vi "AlignMini.vi"() -> ()   [LabVIEW 2019]
uses:
  <vilib>/userDefined/High Color/IMAQdx.ctl
  <vilib>/vision/driver/NI_Vision_Acquisition_Software.lvlib
  <vilib>/vision/NI_Vision_Development_Module.lvlib
panel:
  in  "Second Fiducial in View?":bool
  out "Image Out":T1(plugin-control)
  in  "Fiducial 1":bool
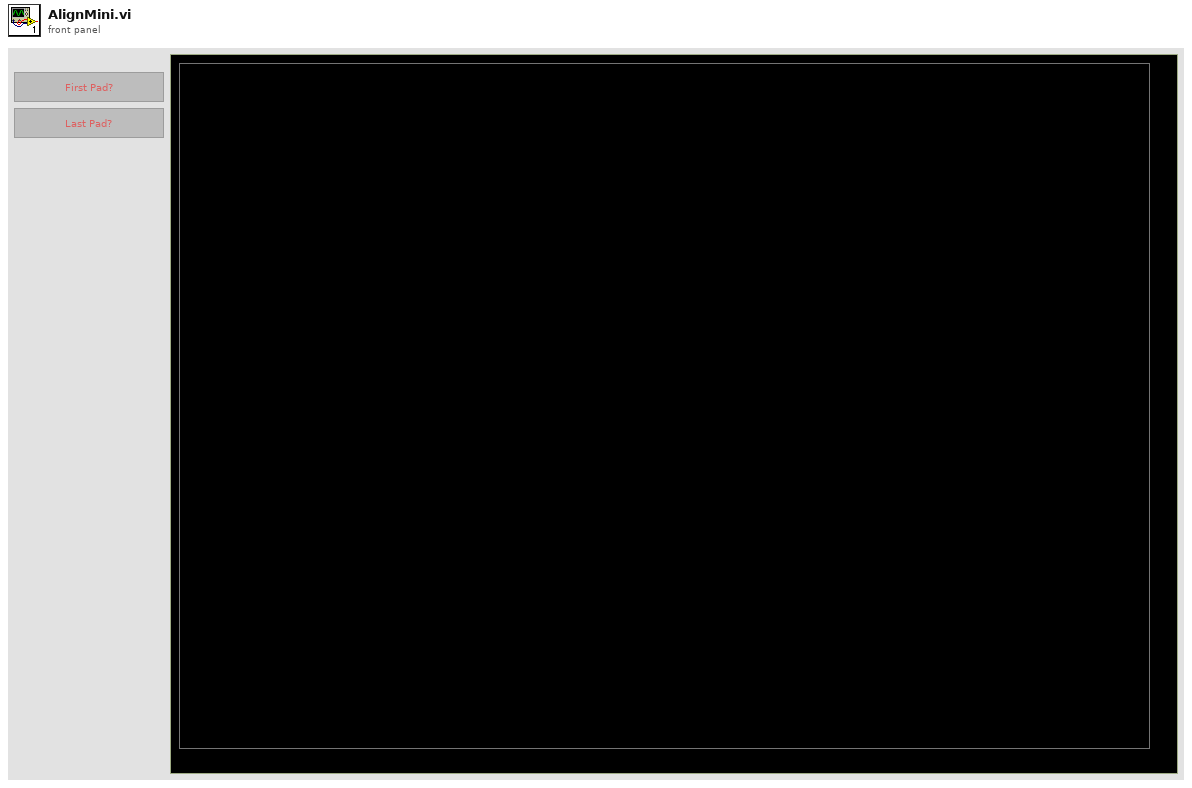
[diagram p1: front panel]
types:
  T1 = typedef "IMAQ Image.ctl" = refnum<image>
  T2 = enum8{"Enabled", "Disabled", "Disabled and Grayed Out"}
  T3 = typedef "Image Type" = u32
  T4 = typedef "IMAQdx.ctl" = refnum<k21>
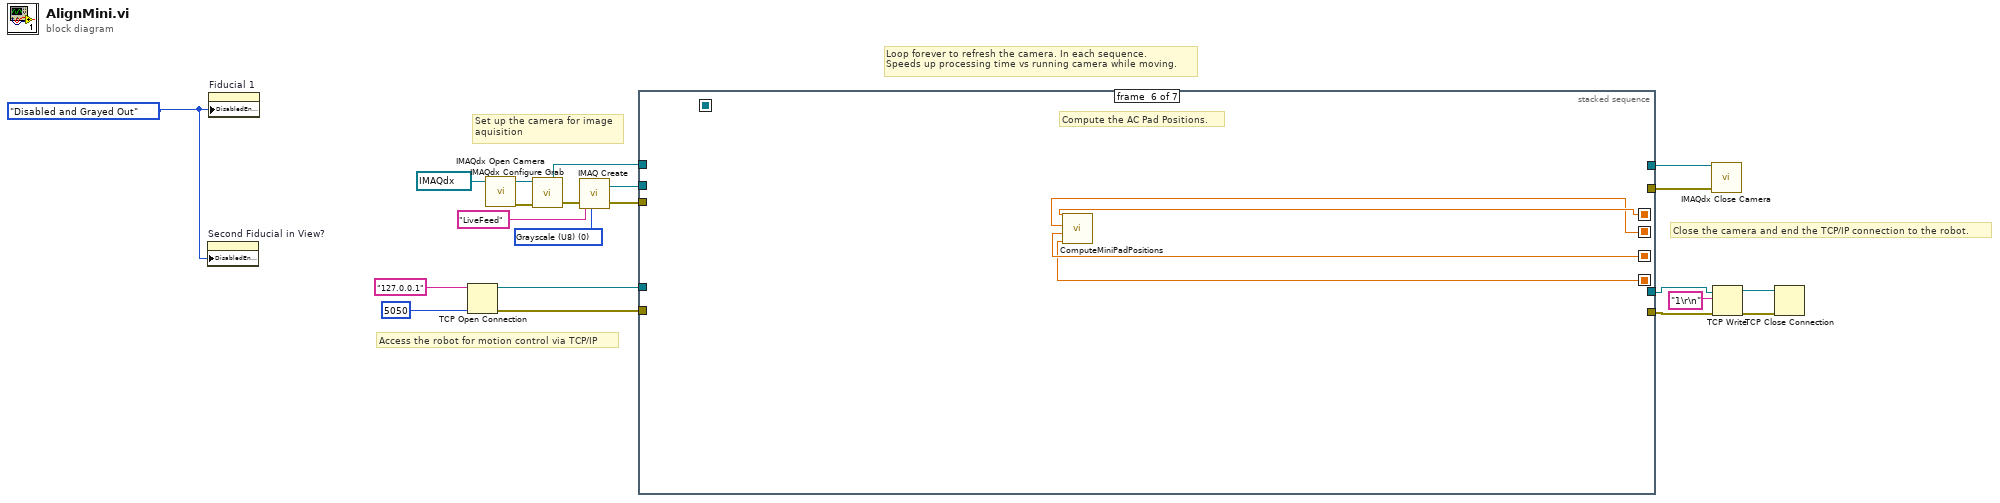
[diagram p0: block diagram]
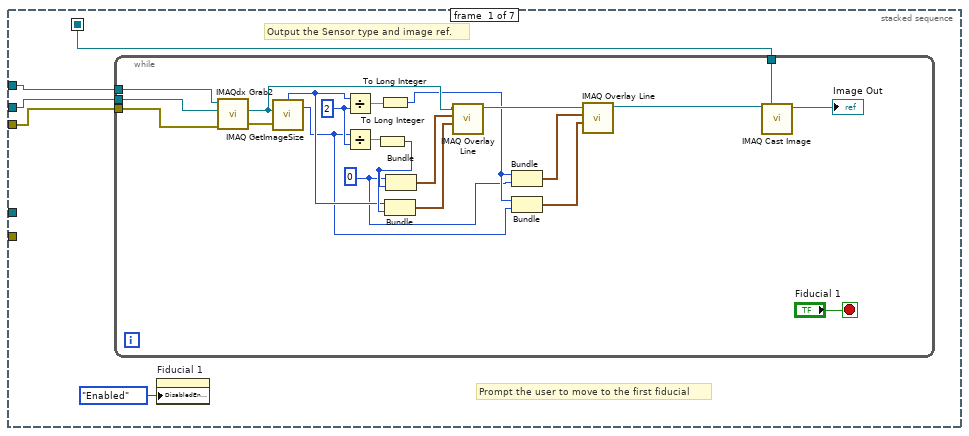
[diagram p2: hidden frame]
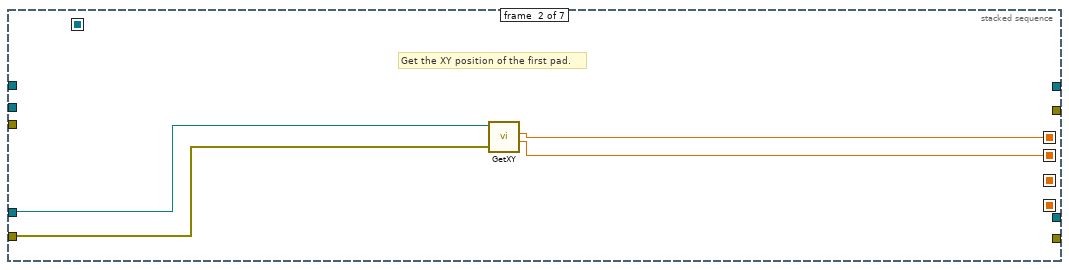
[diagram p3: hidden frame]
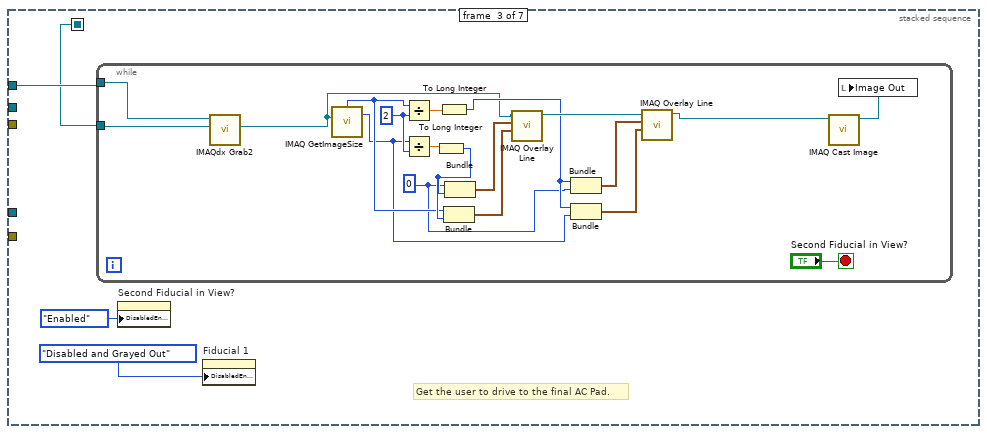
[diagram p4: hidden frame]
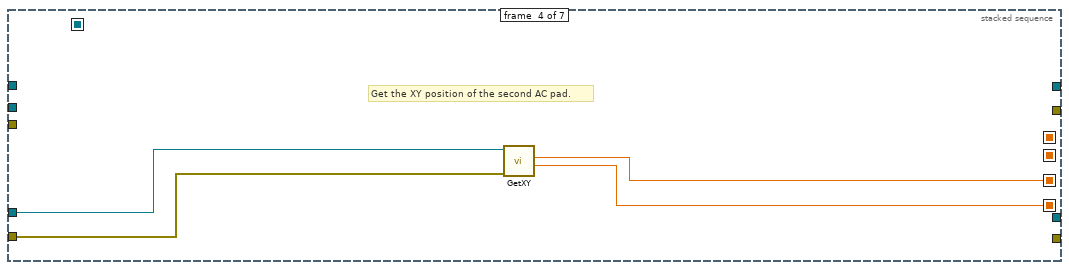
[diagram p5: hidden frame]
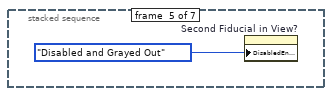
[diagram p6: hidden frame]
diagram:
  w1 = T2."Disabled and Grayed Out" ("Disabled")
  w11 = T3 0 items=["Grayscale (U8)", "Grayscale (I16)", "Grayscale (SGL)", "Complex (CSG)", "RGB (U32)", "HSL (U32)", "RGB (U64)", "Grayscale (U16)"] ("Image Type")
  # "Close the camera and end the TCP/IP connection to the robot."
  # "Access the robot for motion control via TCP/IP"
  # "Loop forever to refresh the camera. In each sequence. \nSpeeds up processing time vs running camera while moving."
  # "Set up the camera for image \naquisition"
  n1 = property on="Second Fiducial in View?" class="Bool"("DisabledEnum"=w1) -> ()  [unwired: 2 in, 2 out]
  n2 = property on="Fiducial 1" class="Bool"("DisabledEnum"=w1) -> ()  [unwired: 2 in, 2 out]
  n3 = TCP Open Connection(address="127.0.0.1", remote port or service name=u16 5050) -> (connection ID=w8:refnum<k5>, error out=w7:errorcluster)  [unwired: 3 in]
  n4 = call <vilib>:"IMAQdx Open Camera.vi"("Session In"=T4 "cam0") -> ("error out"=w19:errorcluster, "Session Out"=w20:T4)  [unwired: 9 in]
  n5 = call <vilib>:"IMAQdx Configure Grab.vi"("error in"=w19, "Session In"=w20) -> ("error out"=w17:errorcluster, "Session Out"=w16:T4)  [unwired: 8 in]
  n6 = call "IMAQ Create"("Image Name"="LiveFeed", "Image Type"=w11, "error in (no error)"=w17) -> ("New Image"=w15:T1, "error out"=w14:errorcluster)  [unwired: 2 in]
  n7 = stacked-sequence {
    seq-local: [w23 _ _ _ _ _ _] -> [_ _ w54 _ _ _ _]
    seq-local: [_ _ _ w76 _ _ _] -> [_ _ _ _ _ w81 _]
    seq-local: [_ _ _ w75 _ _ _] -> [_ _ _ _ _ w80 _]
    seq-local: [_ w49 _ _ _ _ _] -> [_ _ _ _ _ w83 _]
    seq-local: [_ w48 _ _ _ _ _] -> [_ _ _ _ _ w82 _]
    tunnel: w16 -> [w26 _ w55 _ _ _ w86]
    tunnel: w15 -> [w25 _ _ _ _ _ _]
    tunnel: w14 -> [w24 _ _ _ _ _ w87]
    tunnel: [_ _ _ _ _ _ w87] -> w13
    tunnel: [_ _ _ _ _ _ w86] -> w12
    tunnel: w8 -> [_ w51 _ w78 _ _ w85]
    tunnel: [_ _ _ _ _ _ w85] -> w5
    tunnel: [_ _ _ _ _ _ w84] -> w6
    tunnel: w7 -> [_ w50 _ w77 _ _ w84]
    frame #0 {
      # "Output the Sensor type and image ref."
      # "Prompt the user to move to the first fiducial"
      n8 = while {
        tunnel: w26 -> [w46]
        tunnel: w24 -> [w45]
        tunnel: w25 -> [w44]
        tunnel: [w43] -> w23
        stop <- "Fiducial 1" stop-if-true
        w29 = 0
        w41 = 2 ("y")
        n9 = call <vilib>:"IMAQdx Grab2.vi"("error in"=w45, "Image In"=w44, "Session In"=w46) -> ("error out"=w42:errorcluster, "Image Out"=w35:T1)  [unwired: 5 in, 2 out]
        n10 = call "IMAQ GetImageSize"("Image"=w35, "error in (no error)"=w42) -> ("Y Resolution"=w28:i32, "X Resolution"=w36:i32)  [unwired: 2 in, 1 out]
        n11 = Divide(x=w36, y=w41) -> (x/y=w40:dbl)
        n12 = Divide(x=w28, y=w41) -> (x/y=w39:dbl)
        n13 = To Long Integer(number=w39) -> (32bit integer=w37:i32)
        n14 = To Long Integer(number=w40) -> (32bit integer=w30:i32)
        n15 = Bundle("X Resolution"=w36, w37) -> (w33:cluster{"X Resolution":i32, i32})  [unwired: 1 in]
        n16 = Bundle(w29, w37) -> (w38:cluster{i32, i32})  [unwired: 1 in]
        n17 = call "IMAQ Overlay Line"("End Point"=w33, "Start Point"=w38, "Image"=w35) -> ("Image Out"=w34:T1)  [unwired: 3 in, 5 out]
        n18 = Bundle(w30, w29) -> (w32:cluster{i32, i32})  [unwired: 1 in]
        n19 = Bundle(w30, "Y Resolution"=w28) -> (w31:cluster{i32, "Y Resolution":i32})  [unwired: 1 in]
        n20 = call "IMAQ Overlay Line"("End Point"=w31, "Start Point"=w32, "Image"=w34) -> ("Image Out"=w27:T1)  [unwired: 3 in, 5 out]
        n21 = call "IMAQ Cast Image"("Image Src"=w27) -> ("Image Dst Out"=w43:T1)  [unwired: 9 in, 1 out]
        "Image Out" <- w43
      }
      n22 = property on="Fiducial 1" class="Bool"("DisabledEnum"=T2."Enabled" ("Disabled")) -> ()  [unwired: 2 in, 2 out]
    }
    frame #1 {
      # "Get the XY position of the first pad."
      n23 = call "GetXY.vi"("error in (no error)"=w50, "connection ID"=w51) -> ("Y"=w48:dbl, "X"=w49:dbl)  [unwired: 6 in, 2 out]
    }
    frame #2 {
      # "Get the user to drive to the final AC Pad."
      n24 = while {
        tunnel: w54 -> [w73]
        tunnel: w55 -> [w72]
        stop <- "Second Fiducial in View?" stop-if-true
        w59 = 0
        w70 = 2 ("y")
        n25 = call <vilib>:"IMAQdx Grab2.vi"("Image In"=w73, "Session In"=w72) -> ("Image Out"=w57:T1)  [unwired: 6 in, 3 out]
        n26 = call "IMAQ GetImageSize"("Image"=w57) -> ("Y Resolution"=w58:i32, "X Resolution"=w65:i32)  [unwired: 3 in, 1 out]
        n27 = Divide(x=w65, y=w70) -> (x/y=w69:dbl)
        n28 = Divide(x=w58, y=w70) -> (x/y=w68:dbl)
        n29 = To Long Integer(number=w68) -> (32bit integer=w66:i32)
        n30 = To Long Integer(number=w69) -> (32bit integer=w60:i32)
        n31 = Bundle("X Resolution"=w65, w66) -> (w63:cluster{"X Resolution":i32, i32})  [unwired: 1 in]
        n32 = Bundle(w59, w66) -> (w67:cluster{i32, i32})  [unwired: 1 in]
        n33 = call "IMAQ Overlay Line"("End Point"=w63, "Start Point"=w67, "Image"=w57) -> ("Image Out"=w64:T1)  [unwired: 3 in, 5 out]
        n34 = Bundle(w60, w59) -> (w62:cluster{i32, i32})  [unwired: 1 in]
        n35 = Bundle(w60, "Y Resolution"=w58) -> (w61:cluster{i32, "Y Resolution":i32})  [unwired: 1 in]
        n36 = call "IMAQ Overlay Line"("End Point"=w61, "Start Point"=w62, "Image"=w64) -> ("Image Out"=w56:T1)  [unwired: 3 in, 5 out]
        n37 = call "IMAQ Cast Image"("Image Src"=w56) -> ("Image Dst Out"=w71:T1)  [unwired: 9 in, 1 out]
        n38 = local write "Image Out"(w71) -> ()
      }
      n39 = property on="Second Fiducial in View?" class="Bool"("DisabledEnum"=T2."Enabled" ("Disabled")) -> ()  [unwired: 2 in, 2 out]
      n40 = property on="Fiducial 1" class="Bool"("DisabledEnum"=T2."Disabled and Grayed Out" ("Disabled")) -> ()  [unwired: 2 in, 2 out]
    }
    frame #3 {
      # "Get the XY position of the second AC pad."
      n41 = call "GetXY.vi"("error in (no error)"=w77, "connection ID"=w78) -> ("Y"=w75:dbl, "X"=w76:dbl)  [unwired: 6 in, 2 out]
    }
    frame #4 {
      n42 = property on="Second Fiducial in View?" class="Bool"("DisabledEnum"=T2."Disabled and Grayed Out" ("Disabled")) -> ()  [unwired: 2 in, 2 out]
    }
    frame #5 {
      # "Compute the AC Pad Positions."
      n43 = call "ComputeMiniPadPositions.vi"("X1"=w83, "Y1"=w82, "X2"=w81, "Y2"=w80) -> ()  [unwired: 7 in]
    }
    frame #6 {
      # "Close connections"
    }
  }
  n44 = call <vilib>:"IMAQdx Close Camera.vi"("error in"=w13, "Session In"=w12) -> ()  [unwired: 9 in, 1 out]
  n45 = TCP Write(connection ID=w5, data in="1\r\n", error in (no error)=w6) -> (connection ID out=w3:refnum<k5>, error out=w4:errorcluster)  [unwired: 1 in, 1 out]
  n46 = TCP Close Connection(connection ID=w3, error in (no error)=w4) -> ()  [unwired: 1 in, 2 out]
